vi "Datasheet Process Parameters.vi"(4 "Report Field Display Names":T10, 5 "Template Record":T4, 6 "System or ALL Combined Fields":T1[](array[typedef]), 7 "Preview?":bool, 8 "error in (no error)":errorcluster, 9 "Runs for this plot":T5[](array[typedef]), 10 "Parameters":T8, 11 "Connection Refnum":T9) -> (0 "error out":errorcluster, 2 "Parameters":T8, 3 "Connection Refnum":T9)   [LabVIEW 2011]
uses:
  Datasheet Field Display Names.ctl
  SI.LIB/ODBC/SQL Controls/Connection Refnum.ctl
  Addons/internet/utils/keyedarr.llb/Keyed Array.ctl
  TDMS/TDMS File.ctl
  TDMS/TDMS Run.ctl
  TDMS/TDMS Channel (Sxx).ctl
  database/Fields/Field Record.ctl
  database/Fields/Field DataTypes.ctl
  database/Fields/Field NextItem.ctl
  database/Templates/Template Record.ctl
  Addons/internet/utils/strutil.llb/Case Matching.ctl
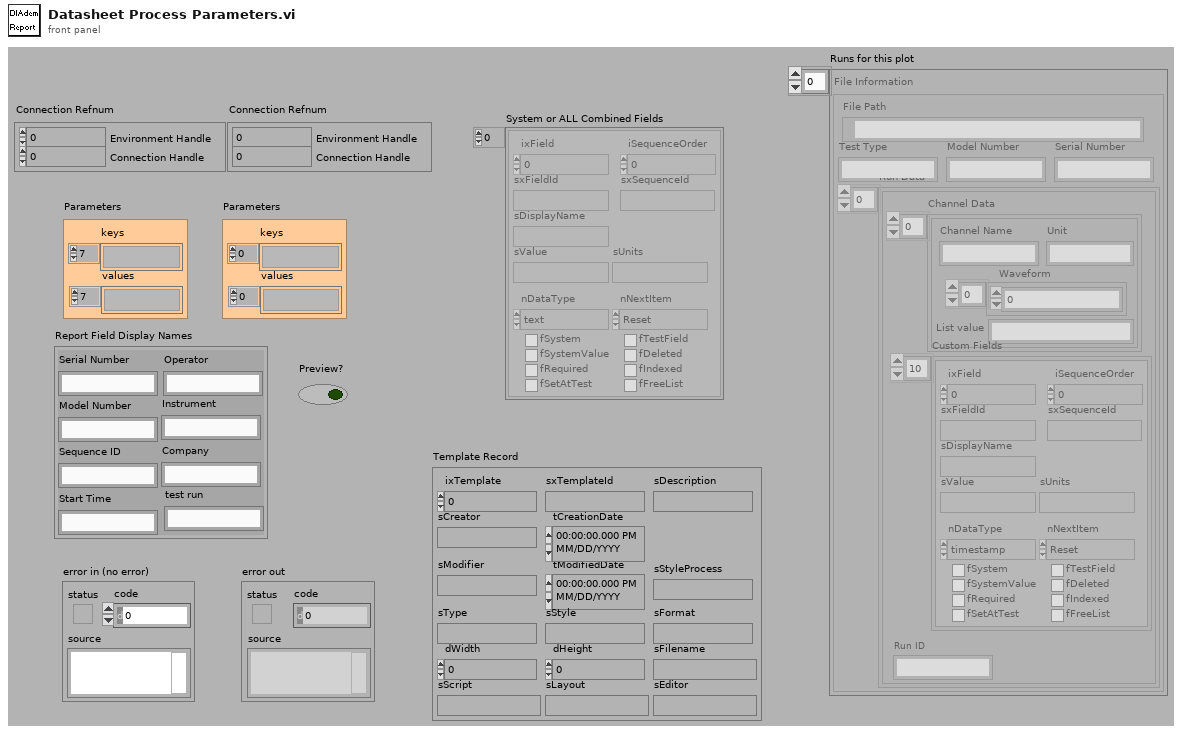
[diagram p1: front panel]
types:
  T1 = typedef "Field Record.ctl" = cluster{"ixField":i32, "iSequenceOrder":i32, "sxFieldId":string, "sxSequenceId":string, "sDisplayName":string, "sValue":string, "sUnits":string, "nDataType":T2, "nNextItem":T3, "fSystem":bool, "fSystemValue":bool, "fRequired":bool, "fSetAtTest":bool, "fTestField":bool, "fDeleted":bool, "fIndexed":bool, "fFreeList":bool}
  T2 = typedef "Field DataTypes.ctl" = enum32{"text", "numeric", "list", "timestamp", "boolean"}
  T3 = typedef "Field NextItem.ctl" = enum32{"Reset", "Retain", "Auto-Increment"}
  T4 = typedef "Template Record.ctl" = cluster{"ixTemplate":i32, "sxTemplateId":string, "sDescription":string, "sCreator":string, "tCreationDate":timestamp, "sModifier":string, "tModifiedDate":timestamp, "sType":string, "sStyle":string, "sFormat":string, "dWidth":dbl, "dHeight":dbl, "sFilename":string, "sScript":string, "sLayout":string, "sEditor":string, "sStyleProcess":string}
  T5 = typedef "TDMS File.ctl" = cluster{"File Path":path, "Run Data":T6[], "Serial Number":string, "Model Number":string, "Test Type":string}
  T6 = typedef "TDMS Run.ctl" = cluster{"Channel Data":T7[], "Custom Fields":T1[], "Run ID":string}
  T7 = typedef "TDMS Channel (Sxx).ctl" = cluster{"Channel Name":string, "Waveform":dbl[], "Unit":string, "List value":string}
  T8 = typedef "Keyed Array.ctl" = cluster{"keys":string[], "values":string[]}
  T9 = typedef "Connection Refnum.ctl" = cluster{"Environment Handle":i32, "Connection Handle":i32}
  T10 = typedef "DATASHEET Field Display Names.ctl" = cluster{"Serial Number":string, "Model Number":string, "Sequence ID":string, "Start Time":string, "Instrument":string, "Company":string, "Operator":string, "test run":string}
  T11 = typedef "Case Matching.ctl" = enum16{"a != A", "a == A", "system"}
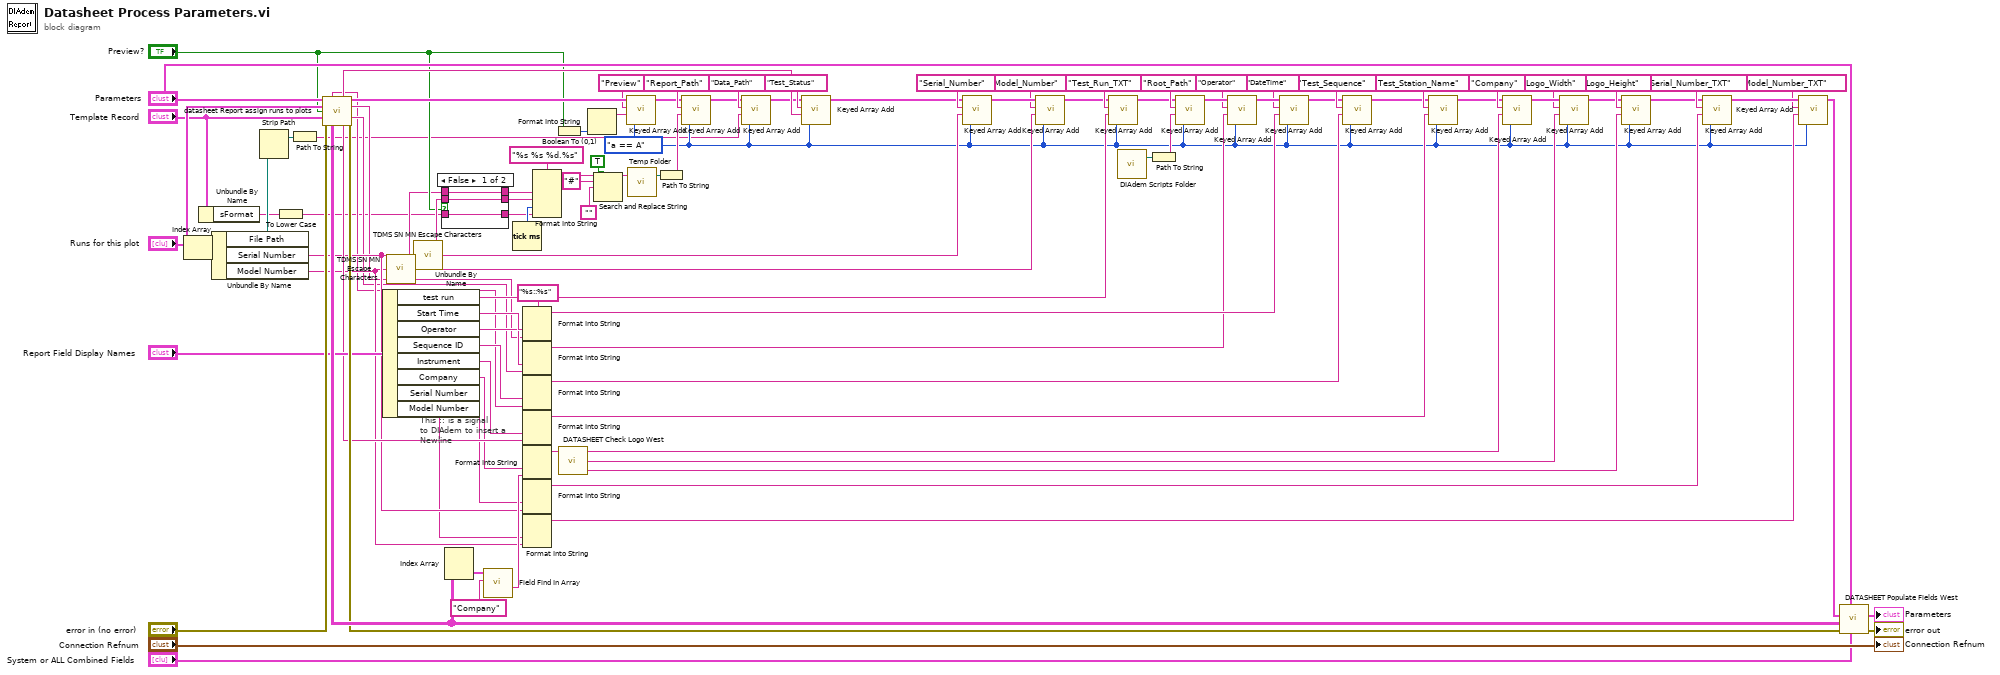
[diagram p0: block diagram]
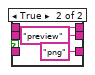
[diagram p2: hidden frame]
diagram:
  w31 = "%s::%s" ("format string")
  w8 = Case_Matching."a == A" ("case matching (sensitive)")
  # "This :: is a signal \nto DIAdem to insert a\nNewline"
  n1 = Index Array(array="Runs for this plot") -> (element=w81:T5)  [unwired: 1 in]
  n2 = Unbundle By Name("Template Record") -> ("sFormat"=w3:string)
  n3 = Unbundle By Name(w81) -> ("File Path"=w7:path, "Serial Number"=w17:string, "Model Number"=w16:string)
  n4 = Strip Path(path=w7) -> (stripped path=w6:path)  [unwired: 1 out]
  n5 = To Lower Case(string=w3) -> (all lower case string=w2:string)
  n6 = Path To String(path=w6) -> (string=w5:string)
  n7 = call "datasheet Report assign runs to plots.vi"("Parameters"="Parameters", "Runs for this plot"="Runs for this plot", "Preview?"="Preview?", "Template Record"="Template Record", "error in (no error)"="error in (no error)") -> ("sequence"=w13:string, "test status"=w73:string, "Parameters"=w68:T8, "time stamp"=w15:string, "operator"=w14:string, "Custom Fields"=w70:T1[][], "test station"=w21:string, "error out"=w69:errorcluster)  [unwired: 3 out]
  n8 = Unbundle By Name("Report Field Display Names") -> ("test run"=w42:string, "Start Time"=w33:string, "Operator"=w24:string, "Sequence ID"=w23:string, "Instrument"=w22:string, "Company"=w20:string, "Serial Number"=w18:string, "Model Number"=w12:string)
  n9 = call "TDMS SN MN Escape Characters.vi"("string"=w16) -> ("url-encoded string"=w34:string)
  n10 = call "TDMS SN MN Escape Characters.vi"("string"=w17) -> ("url-encoded string"=w57:string)
  n11 = case shown="False" "Preview?" {
    tunnel: [w102 "png" ("format string")] -> w38
    tunnel: [w103 w106] -> w37
    tunnel: [w104 w106] -> w36
    tunnel: w34 -> [w104 _]
    tunnel: w57 -> [w103 _]
    tunnel: w2 -> [w102 _]
    frame False {
    }
    frame True {
      w106 = "preview" ("format string")
    }
  }
  n12 = Index Array(array=w70) -> (element=w56:T1[])  [unwired: 2 in]
  n13 = call "Field Find In Array.vi"("FieldID or Display Name(\"\")"="Company" ("format string"), "Field Array"=w56) -> ("sValue"=w19:string)  [unwired: 1 in, 8 out]
  n14 = Tick Count (ms)() -> (millisecond timer value=w39:u32)
  n15 = Format Into String(format string=w31, w33, w15) -> (resulting string=w32:string)  [unwired: 2 in, 1 out]
  n16 = Format Into String(format string=w31, w24, w14) -> (resulting string=w30:string)  [unwired: 2 in, 1 out]
  n17 = Format Into String(format string=w31, w23, w13) -> (resulting string=w29:string)  [unwired: 2 in, 1 out]
  n18 = Format Into String(format string=w31, w22, w21) -> (resulting string=w28:string)  [unwired: 2 in, 1 out]
  n19 = Format Into String(format string=w31, w20, w19) -> (resulting string=w27:string)  [unwired: 2 in, 1 out]
  n20 = Format Into String(format string=w31, w18, w17) -> (resulting string=w26:string)  [unwired: 2 in, 1 out]
  n21 = Format Into String(format string=w31, w12, w16) -> (resulting string=w25:string)  [unwired: 2 in, 1 out]
  n22 = Format Into String(format string="%s %s %d.%s", w36, w37, w39, w38) -> (resulting string=w35:string)  [unwired: 2 in, 1 out]
  n23 = Boolean To (0,1)(Boolean="Preview?") -> (0, 1=w46:i16)
  n24 = call "DATASHEET Check Logo West.vi"("Company_ID_Txt"=w27) -> ("Insertion Height"=w58:string, "Insertion Width"=w62:string, "Company_ID_Txt"=w94:string)  [unwired: 2 out]
  n25 = Format Into String(w46) -> (resulting string=w45:string)  [unwired: 3 in, 1 out]
  n26 = Search and Replace String(replace all?=TRUE ("replace all? (F)"), input string=w35, search string="#", replace string="") -> (result string=w50:string)  [unwired: 4 in, 3 out]
  n27 = call "Keyed Array Add.vi"("case matching (sensitive)"=w8, "value"=w45, "key"="Preview" ("format string"), "array in"=w68) -> ("array out"=w67:T8)  [unwired: 3 out]
  n28 = call "Temp Folder.vi"("Relative Path (\"\")"=w50) -> ("Temp Folder"=w77:path)  [unwired: 2 in]
  n29 = Path To String(path=w77) -> (string=w83:string)
  n30 = call "Keyed Array Add.vi"("case matching (sensitive)"=w8, "value"=w83, "key"="Report_Path" ("format string"), "array in"=w67) -> ("array out"=w10:T8)  [unwired: 3 out]
  n31 = call "Keyed Array Add.vi"("case matching (sensitive)"=w8, "value"=w5, "key"="Data_Path" ("format string"), "array in"=w10) -> ("array out"=w9:T8)  [unwired: 3 out]
  n32 = call "Keyed Array Add.vi"("case matching (sensitive)"=w8, "value"=w73, "key"="Test_Status" ("format string"), "array in"=w9) -> ("array out"=w1:T8)  [unwired: 3 out]
  n33 = call "Keyed Array Add.vi"("case matching (sensitive)"=w8, "value"=w57, "key"="Serial_Number" ("format string"), "array in"=w1) -> ("array out"=w76:T8)  [unwired: 3 out]
  n34 = call "Keyed Array Add.vi"("case matching (sensitive)"=w8, "value"=w34, "key"="Model_Number" ("format string"), "array in"=w76) -> ("array out"=w53:T8)  [unwired: 3 out]
  n35 = call "Keyed Array Add.vi"("case matching (sensitive)"=w8, "value"=w42, "key"="Test_Run_TXT" ("format string"), "array in"=w53) -> ("array out"=w54:T8)  [unwired: 3 out]
  n36 = call "DIAdem Scripts Folder.vi"() -> ("Scripts Folder"=w101:path)  [unwired: 1 in, 2 out]
  n37 = Path To String(path=w101) -> (string=w84:string)
  n38 = call "Keyed Array Add.vi"("case matching (sensitive)"=w8, "value"=w84, "key"="Root_Path" ("format string"), "array in"=w54) -> ("array out"=w92:T8)  [unwired: 3 out]
  n39 = call "Keyed Array Add.vi"("case matching (sensitive)"=w8, "value"=w30, "key"="Operator" ("format string"), "array in"=w92) -> ("array out"=w86:T8)  [unwired: 3 out]
  n40 = call "Keyed Array Add.vi"("case matching (sensitive)"=w8, "value"=w32, "key"="DateTime" ("format string"), "array in"=w86) -> ("array out"=w87:T8)  [unwired: 3 out]
  n41 = call "Keyed Array Add.vi"("case matching (sensitive)"=w8, "value"=w29, "key"="Test_Sequence" ("format string"), "array in"=w87) -> ("array out"=w85:T8)  [unwired: 3 out]
  n42 = call "Keyed Array Add.vi"("case matching (sensitive)"=w8, "value"=w28, "key"="Test_Station_Name" ("format string"), "array in"=w85) -> ("array out"=w89:T8)  [unwired: 3 out]
  n43 = call "Keyed Array Add.vi"("case matching (sensitive)"=w8, "value"=w94, "key"="Company" ("format string"), "array in"=w89) -> ("array out"=w64:T8)  [unwired: 3 out]
  n44 = call "Keyed Array Add.vi"("case matching (sensitive)"=w8, "value"=w62, "key"="Logo_Width" ("format string"), "array in"=w64) -> ("array out"=w60:T8)  [unwired: 3 out]
  n45 = call "Keyed Array Add.vi"("case matching (sensitive)"=w8, "value"=w58, "key"="Logo_Height" ("format string"), "array in"=w60) -> ("array out"=w59:T8)  [unwired: 3 out]
  n46 = call "Keyed Array Add.vi"("case matching (sensitive)"=w8, "value"=w26, "key"="Serial_Number_TXT" ("format string"), "array in"=w59) -> ("array out"=w96:T8)  [unwired: 3 out]
  n47 = call "Keyed Array Add.vi"("case matching (sensitive)"=w8, "value"=w25, "key"="Model_Number_TXT" ("format string"), "array in"=w96) -> ("array out"=w98:T8)  [unwired: 3 out]
  n48 = call "DATASHEET Populate Fields West.vi"("System or ALL Combined Fields"="System or ALL Combined Fields", "Source Parameters"="Parameters", "error in (no error)"=w69, "Custom Fields"=w70, "Parameters"=w98) -> ("error out"=→"error out":errorcluster, "Parameters 2"=→"Parameters":T8)  [unwired: 2 in, 3 out]
  "Connection Refnum" <- "Connection Refnum"
